vi "Set CellValue.vi"(8 "error in":errorcluster, 10 "CellValue in":refnum<k24>, 11 "Cell in":refnum<k24>) -> (0 "error out":errorcluster, 2 "CellValue out":refnum<k24>, 3 "Cell out":refnum<k24>)   [LabVIEW 2019, in "Open Xml.lvlib"]
uses:
  Open Xml.lvlib
  D:/git/Open-Xml-LabVIEW/Source/DocumentFormat.OpenXml.dll
  DocumentFormat.OpenXml.dll
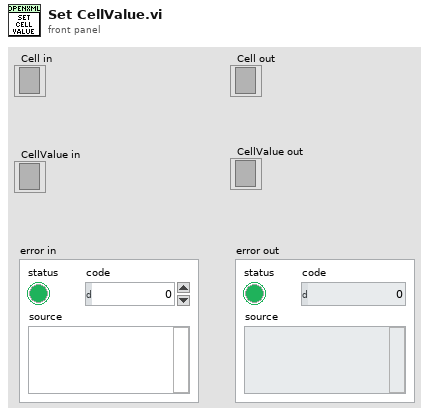
[diagram p1: front panel]
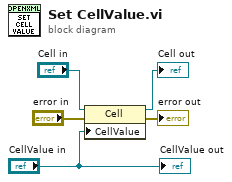
[diagram p0: block diagram]
diagram:
  n1 = property class="Cell"(reference="Cell in", error in="error in", "CellValue"="CellValue in") -> (reference out=→"Cell out":refnum<k24>, error out=→"error out":errorcluster)
  "CellValue out" <- "CellValue in"
